vi "LookupTable-Rhom.vi"(1 "Lookup index":u64, 2 "file path (dialog if empty)":path=path "C:/Users/Lexa/DevProjects/Prometheus/Scalable packed voxel mapping/LookupTable-Rhombohedral.csv") -> (0 "subarray":i64[](array[numeric]))   [LabVIEW 2020]
uses:
  <vilib>/Utility/file.llb/Read Delimited Spreadsheet (I64).vi
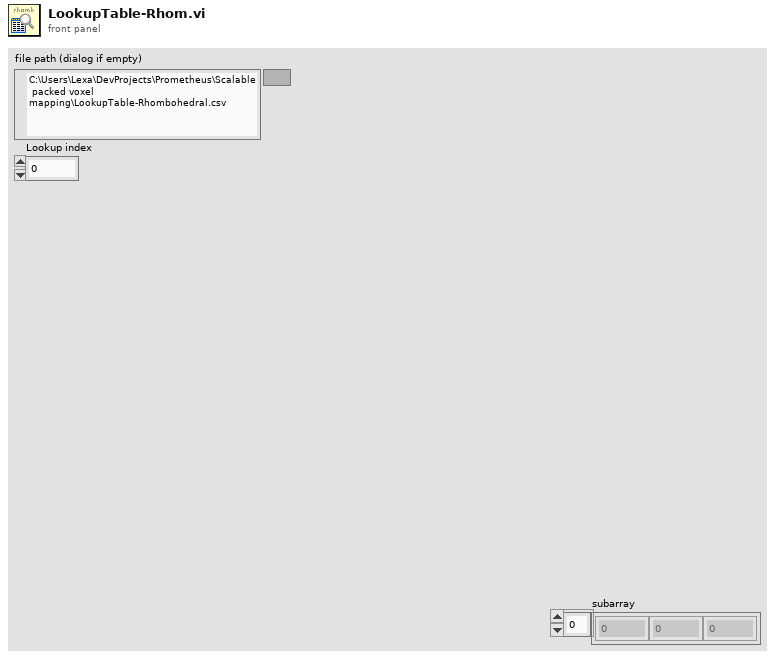
[diagram p1: front panel]
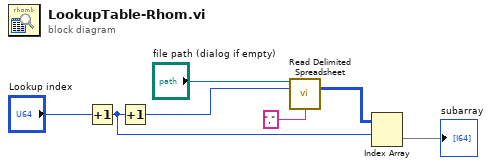
[diagram p0: block diagram]
diagram:
  n1 = Increment(x="Lookup index") -> (x+1=w1:u64)
  n2 = Increment(x=w1) -> (x+1=w2:u64)
  n3 = call-poly <vilib>:"Read Delimited Spreadsheet.vi"("file path (dialog if empty)"="file path (dialog if empty)", "number of rows (all:-1)"=w2, "delimiter (\\t)"="," ("delimiter (\\t)")) -> ("all rows"=w5:i64[][])  [unwired: 7 in, 5 out]
  n4 = Index Array(array=w5, index (row)=w1) -> (element=→"subarray":i64[])  [unwired: 1 in]
